vi "SCFGIN.vi"() -> ()   [LabVIEW 2017]
panel:
  out "data in":string
  in  "stop":bool
  in  "port":u16=8888
  in  "address":string="10.5.4.109"
  in  "pin 14":enum16{"input", "output", "disable"}(ring)=enum."disable"
  out "NewVal":enum16{"input", "output", "disable"}(ring)
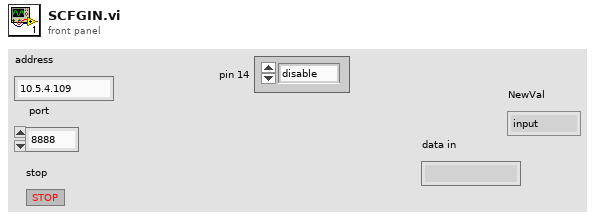
[diagram p1: front panel]
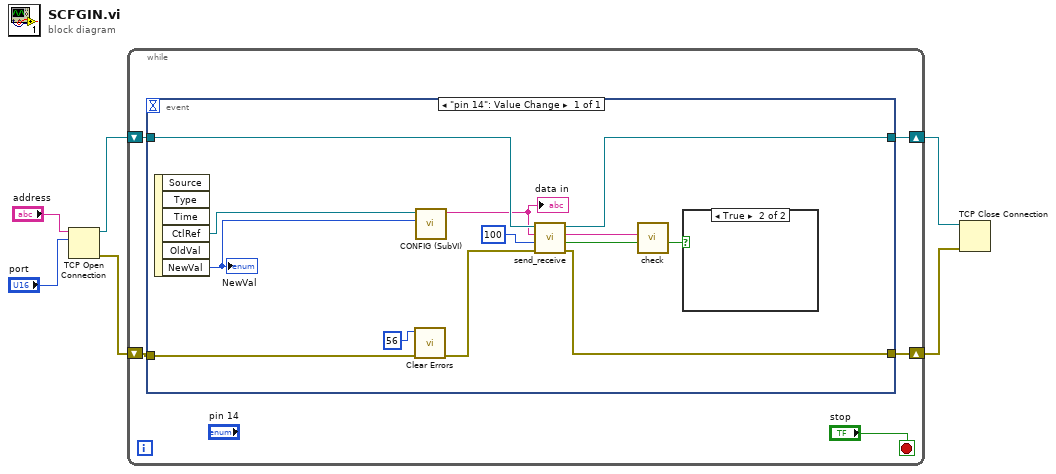
[diagram p0: block diagram]
diagram:
  n1 = TCP Open Connection(address="address", remote port or service name="port") -> (connection ID=w6:refnum<k5>, error out=w5:errorcluster)  [unwired: 3 in]
  n2 = while {
    shift-right: [w9] -> w2
    shift-left: w6 -> [w11]
    shift-right: [w8] -> w1
    shift-left: w5 -> [w10]
    stop <- "stop" stop-if-true
    n3 = event shown="[0] \"pin 14\": Value Change" {
      selector: _ -> [_]
      dyn-events: _ -> [_]
      timeout: _ -> [_]
      tunnel: w11 -> [w24]
      tunnel: w10 -> [w17]
      tunnel: [w23] -> w8
      tunnel: [w22] -> w9
      event "pin 14": Value Change {
        n4 = event-data() -> ("CtlRef"=w14:refnum<vi>, "NewVal"=w13:enum16{"input", "output", "disable"})  [unwired: 1 in, 4 out]
        "NewVal" <- w13
        n5 = call <vilib>:"Clear Errors.vi"("error in (no error)"=w17, "specific error code to clear (0: all)"=56) -> ("error out"=w16:errorcluster)  [unwired: 4 in, 1 out]
        n6 = call "CONFIG (SubVI).vi"("NewVal"=w13, "Enum in"=w14) -> ("String"=w12:string)  [unwired: 9 in]
        "data in" <- w12
        n7 = call "send_receive.vi"("error in (no error)"=w16, "time"=u32 100, "data in"=w12, "connection ID"=w24) -> ("error out"=w23:errorcluster, "Result"=w20:bool, "data out"=w21:string, "connection ID out"=w22:refnum<k5>)  [unwired: 4 in]
        n8 = call "check.vi"("input result"=w20, "input string"=w21) -> ("Result"=w19:bool)  [unwired: 7 in, 2 out]
        n9 = case shown="True" w19 {
          frame False {
          }
          frame True {
          }
        }
      }
    }
  }
  n10 = TCP Close Connection(connection ID=w2, error in (no error)=w1) -> ()  [unwired: 1 in, 2 out]
